vi "viewerFrontEnd.vi"(8 "error in (no error)":errorcluster, 10 "defaultPath":path=path "D:/Data/Labview/BEC Suite/Hal/Channels/Camera/XML Camera Settings/CameraSettings.xml", 11 "CameraSettingsViewer in":refnum<class "andorSettingsViewer.lvclass">) -> (0 "error out":errorcluster, 3 "CameraSettingsViewer out":refnum<class "andorSettingsViewer.lvclass">)   [LabVIEW 2011, in "Views.lvlib" / "Camera.lvlib" / "andorSettingsViewer.lvclass"]
uses:
  andorSettingsViewer.lvclass
  Tools/Filing/FileSystem/FileSystem.lvclass
  Tools/SettingsEventManager/SettingsEventsManager.lvclass
  Tools/SettingsViewer/settingsViewer.lvclass
panel:
  in  "save Current Settings":bool
  in  "Close Settings Mananger":bool
  in  "Load Current Settings":bool
  in  "Load Settings From File":path
  in  "Tab Control":T1(tab)=enum."shift_speeds"
  in  "acquisition_mode":u16(ring)=2 caption="Acquisition Mode" items=["Single Shot"=1, "Accumulative Series"=2, "Kinetic Series"=3, "Fast Kinetic Series"=4, "Run 'till Abort"=5]
  in  "readout_mode":i16(ring)=1 caption="Readout Mode" items=["Full Vertical Binning"=0, "Single Track"=3, "Multi-Track"=1, "Random Track"=2, "Full Resolusion Image"=4]
  in  "subArea_coordinate":i32(listbox) caption="ROI Coordinates of \nBottom left corner"
  in  "vertical_binning":dbl=1.0 caption="Vertical Binning \n(min 0)"
  in  "horizontal_binning":dbl=1.0 caption="Horizontal Binning \n(min 0)"
  in  "subArea_height":dbl=1024.0 caption="ROI and Single Track:\nROI Height"
  in  "subArea_width":dbl=1024.0 caption="ROI Width"
  in  "offset":dbl caption="Single Track:\nOffset"
  in  "number_tracks":i32 caption="Multi Track:\nNumber of Tracks"
  in  "track_positions":i32(listbox) caption="Track Positions"
  in  "fast_kinetic_shift_speed":dbl caption="Fast Kinetic Shift Speed [MHz]"
  in  "horizontal_shift_speed":enum16{"2.5", "1", "0.05"}(ring) caption="Horizontal Shift Speed [MHz]"
  in  "vertical_shift_speed":T2(ring)=enum."44.975" caption="Vertical Shift Speed [mus]"
  in  "fast_kinetic_image_number":dbl=1.0 caption="Number in fast Kinetic Series"
  in  "fast_kinetic_cycle_time":dbl caption="Fast Kinetic Cycle Time"
  in  "accumulative_cycle_time":dbl caption="Accumulative Cycle Time"
  in  "kinetic_cycle_time":dbl caption="Kinetic Cycle Time"
  in  "accumulation_image_number":dbl=1.0 caption="Number of Accumulations"
  in  "kinetic_image_number":dbl=1.0 caption="Number in Kinetic Series"
  in  "mode":enum16{"Automatic", "Hold Open", "Hold Closed"}(ring) caption="Shutter Mode"
  in  "open_time":dbl=20.0 caption="Shutter Open Time"
  in  "close_time":dbl=20.0 caption="Shutter Close Time"
  in  "exposure_time":dbl=0.02 caption="Exposure Time [s]"
  out "start_trigger":string caption="Trigger Channel"
  in  "trigger_mode":u16(ring) caption="Trigger Mode" items=["Internal"=0, "External"=1, "External Start"=6]
  in  "fast_trigger":bool caption="Fast Triggering"
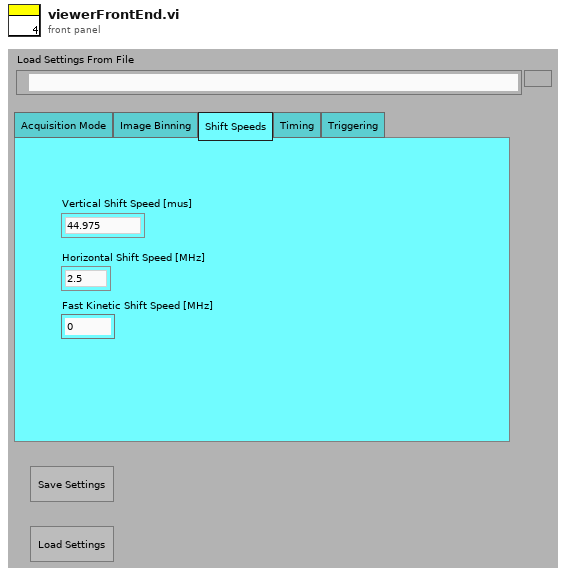
[diagram p1: front panel]
types:
  T1 = enum32{"modes", "image_binning", "shift_speeds", "timing", "triggering"}
  T2 = enum16{"0.525", "0.875", "1.575", "2.975", "5.775", "11.375", "22.575", "44.975"}
  T3 = cluster{"settingsFrontEndEvents":cluster{"loadSettingsFromPath":refnum<user-event>, "lookUpElementEvent":refnum<user-event>, "saveSettings":refnum<user-event>, "loadSettings":refnum<user-event>, "close":refnum<user-event>, "replaceElement":refnum<user-event>, "findParentNodes":refnum<user-event>, "createNode":refnum<user-event>}, "settingBackEndEvents":cluster{"defaultSettingsPathRequest":refnum<user-event>, "searchResultEvent":refnum<user-event>, "settingsSaved":refnum<user-event>, "settingsLoaded":refnum<user-event>, "foundParentNode":refnum<user-event>}}
  T4 = cluster{"loadSettingsFromPath":refnum<user-event>, "lookUpElementEvent":refnum<user-event>, "saveSettings":refnum<user-event>, "loadSettings":refnum<user-event>, "close":refnum<user-event>, "replaceElement":refnum<user-event>, "findParentNodes":refnum<user-event>, "createNode":refnum<user-event>}
  T5 = cluster{"defaultSettingsPathRequest":refnum<user-event>, "searchResultEvent":refnum<user-event>, "settingsSaved":refnum<user-event>, "settingsLoaded":refnum<user-event>, "foundParentNode":refnum<user-event>}
  T6 = enum16{"Number", "String", "NumberArray", "StringArray", "xmlNode"}
  T7 = cluster{"Label.Text":string, string, "DigDisp.Text":string}
  T8 = cluster{"Label.Text":string, string, "RingText.Text":string}
  T9 = typedef "LVPoint32TypeDef.ctl" = cluster{"Horizontal":i32, "Vertical":i32}
  T10 = typedef "LVRowAndColumnTypeDef.ctl" = cluster{"Row":i32, "Column":i32}
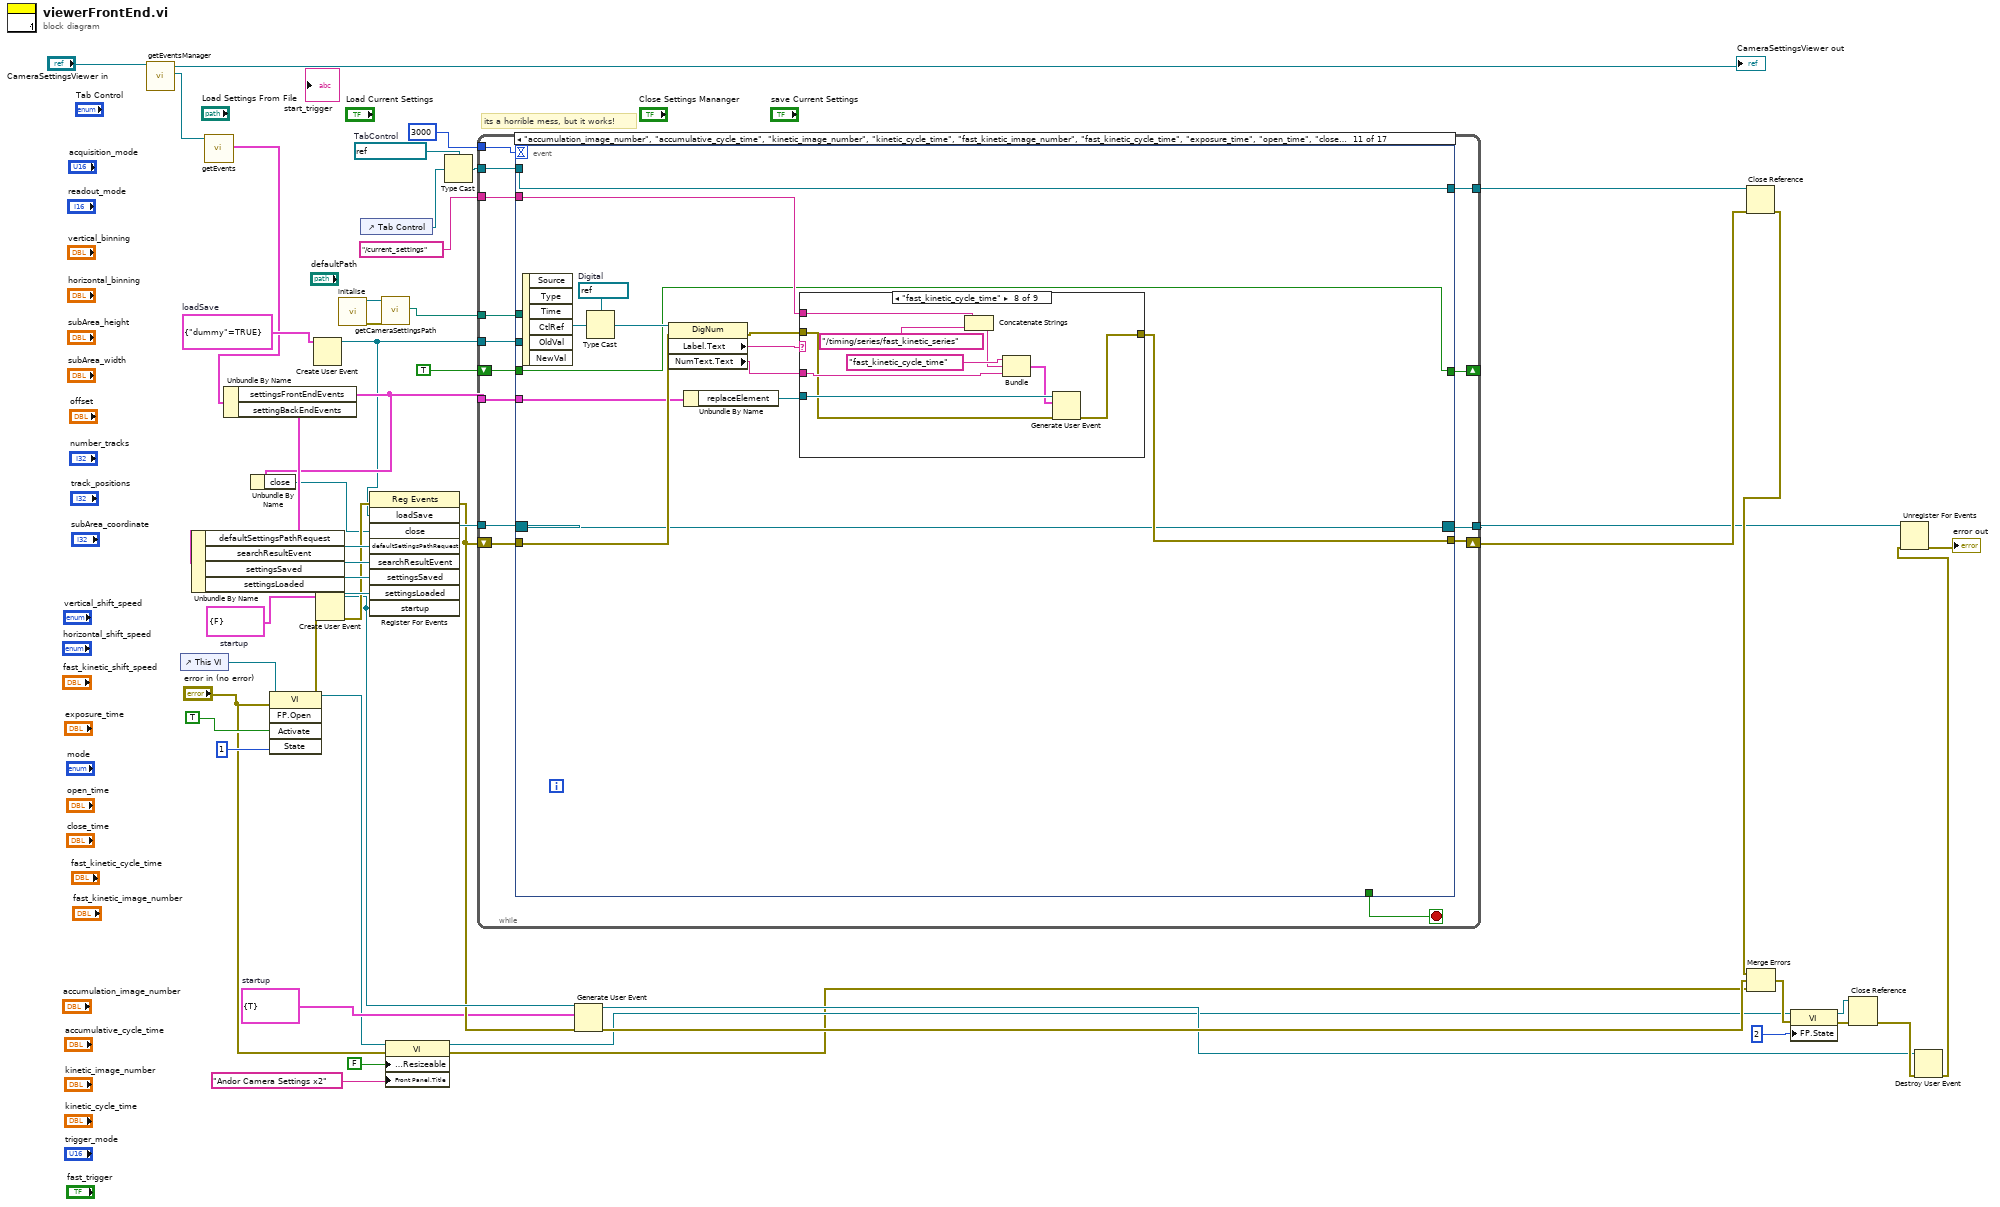
[diagram p0: block diagram]
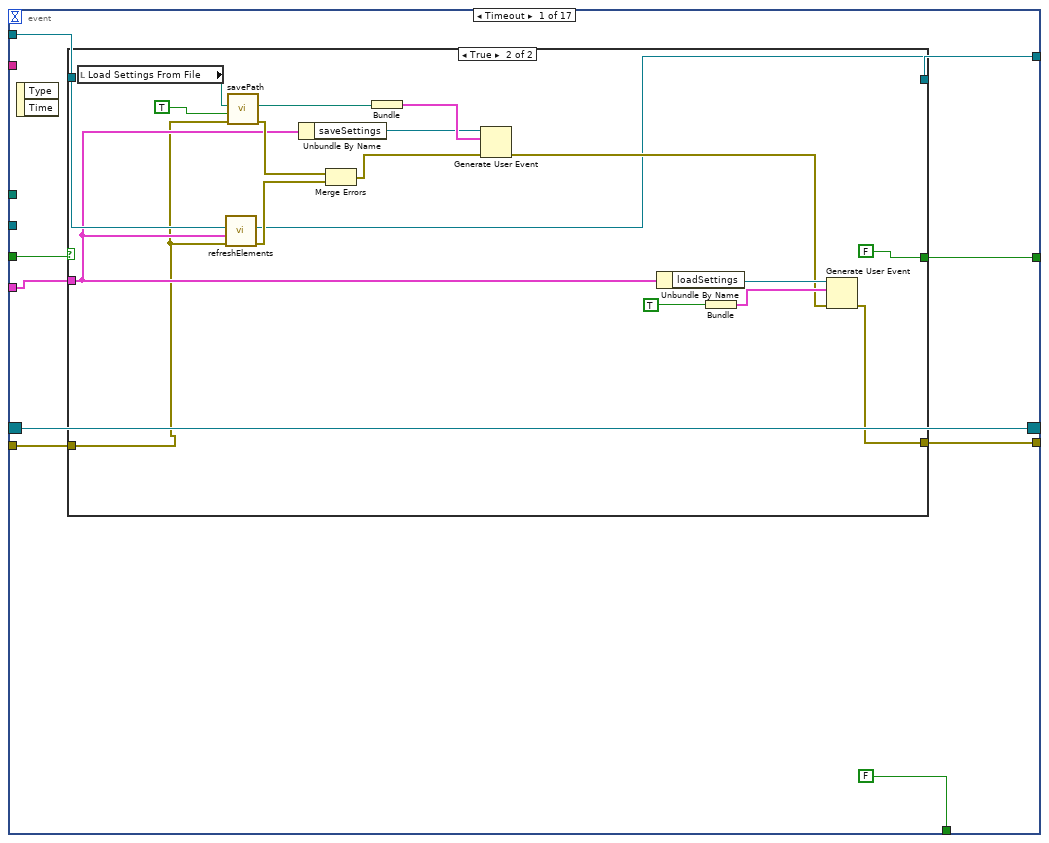
[diagram p2: hidden frame]
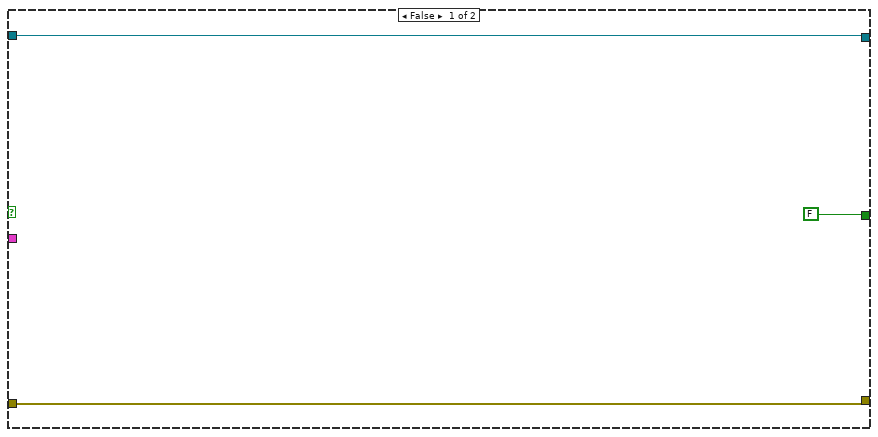
[diagram p3: hidden frame]
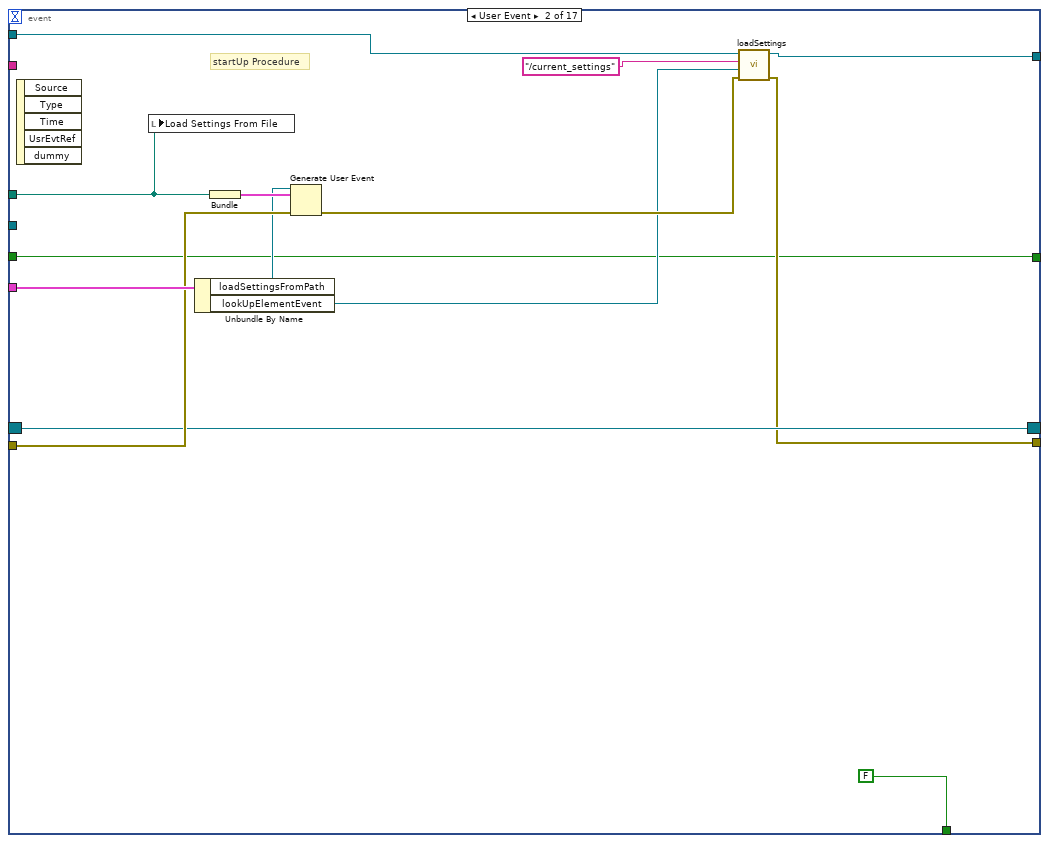
[diagram p4: hidden frame]
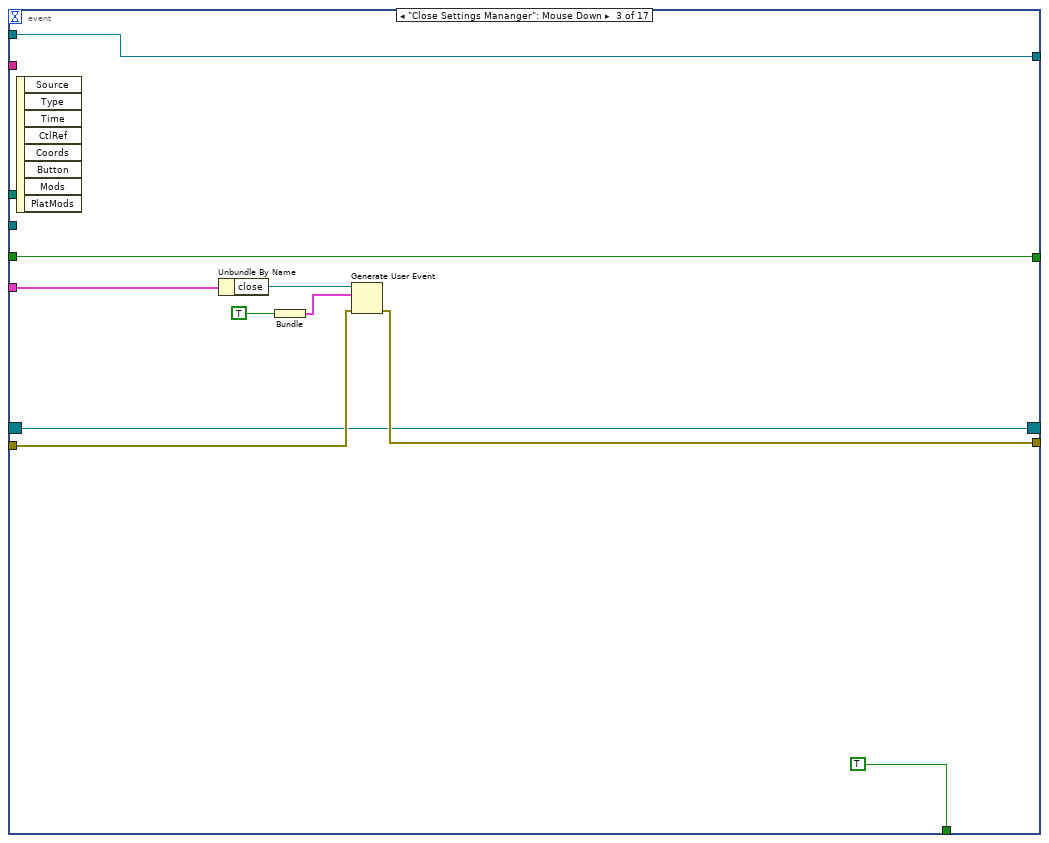
[diagram p5: hidden frame]
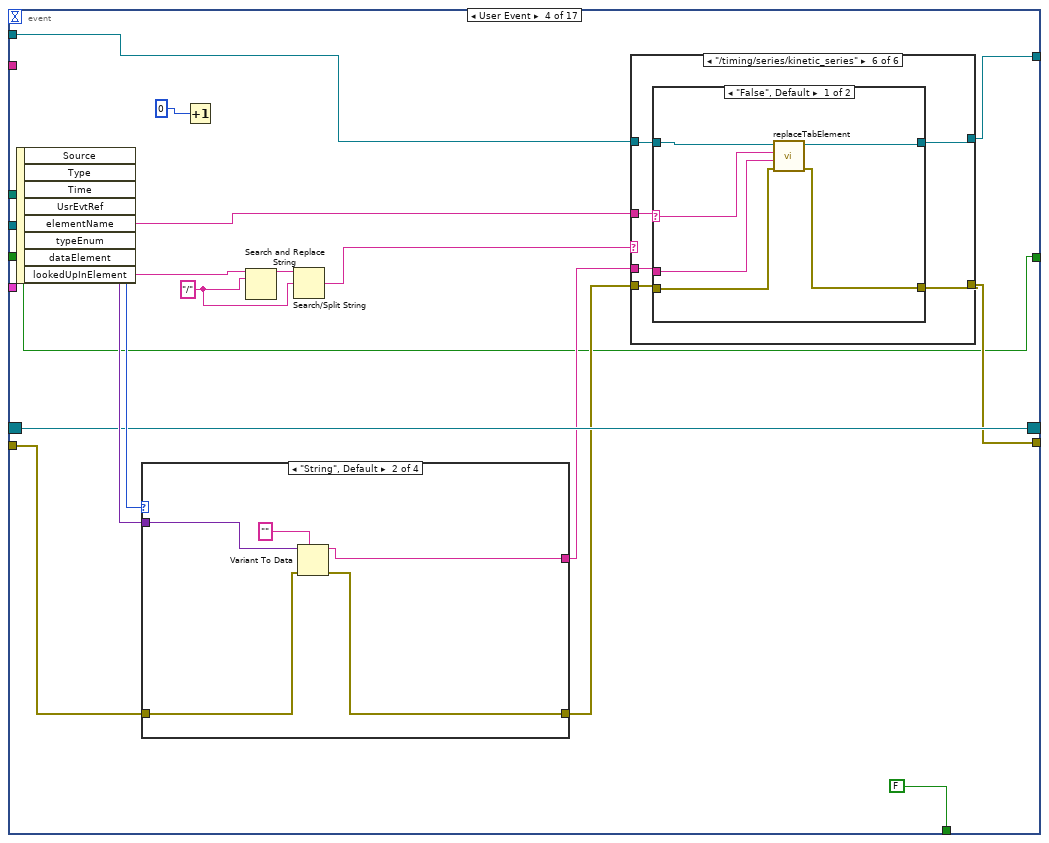
[diagram p6: hidden frame]
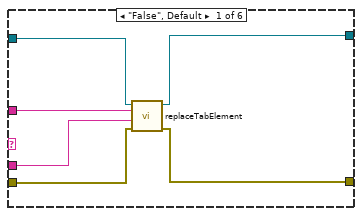
[diagram p7: hidden frame]
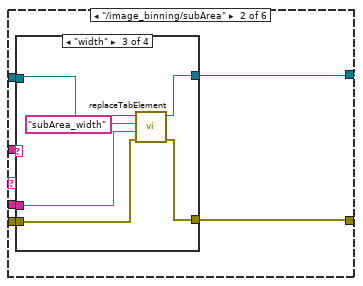
[diagram p8: hidden frame]
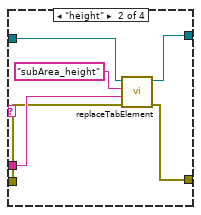
[diagram p10: hidden frame]
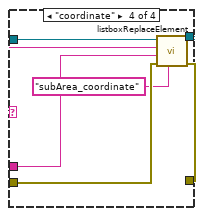
[diagram p11: hidden frame]
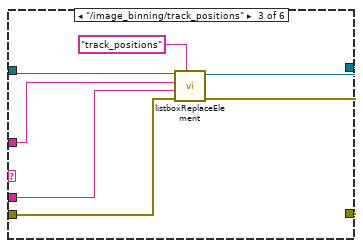
[diagram p12: hidden frame]
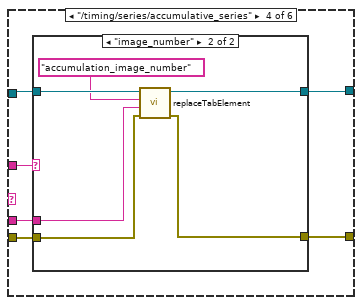
[diagram p13: hidden frame]
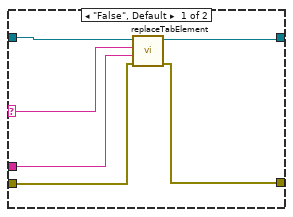
[diagram p14: hidden frame]
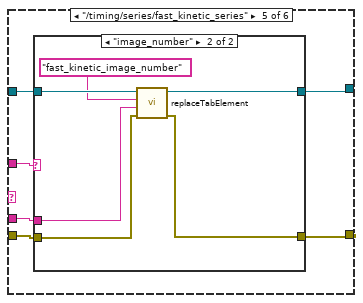
[diagram p15: hidden frame]
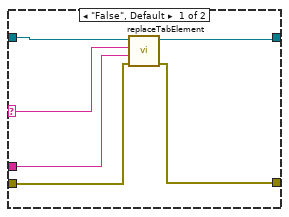
[diagram p16: hidden frame]
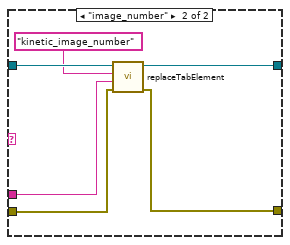
[diagram p17: hidden frame]
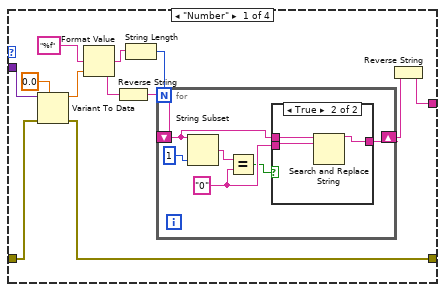
[diagram p18: hidden frame]
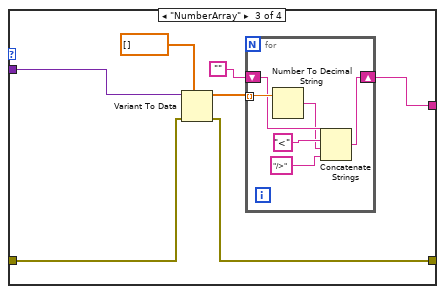
[diagram p20: hidden frame]
diagram:
  w12 = cluster{"dummy":bool} {"dummy"=TRUE}  # loadSave
  w22 = refnum<vi> refnum  # TabControl
  w32 = cluster{"dummy":bool} {"dummy"=TRUE}  # startup
  w36 = cluster{"dummy":bool} {"dummy"=FALSE}  # startup
  # "its a horrible mess, but it works!"
  n1 = call-dynamic "getEventsManager.vi"("SettingsViewer.lvclass in"="CameraSettingsViewer in") -> ("Tools.lvlib:Settings.lvlib:SettingsEventsManager.lvclass"=w8:refnum<class "SettingsEventsManager.lvclass">, "SettingsViewer.lvclass out"=→"CameraSettingsViewer out":refnum<class "andorSettingsViewer.lvclass">)  [unwired: 8 in, 1 out]
  n2 = control-ref of="This VI"() -> (w43:refnum<vi>)
  n3 = call-dynamic "getEvents.vi"("SettingsEventsManager in"=w8) -> ("settingsEvents"=w7:T3)  [unwired: 8 in, 2 out]
  n4 = Unbundle By Name(w7) -> ("settingsFrontEndEvents"=w14:T4, "settingBackEndEvents"=w51:T5)
  n5 = Unbundle By Name(w51) -> ("defaultSettingsPathRequest"=w50:refnum<user-event>, "searchResultEvent"=w49:refnum<user-event>, "settingsSaved"=w48:refnum<user-event>, "settingsLoaded"=w47:refnum<user-event>)
  n6 = Unbundle By Name(w14) -> ("close"=w13:refnum<user-event>)
  n7 = invoke class="VI" method="FP.Open"(reference=w43, error in="error in (no error)", "Activate"=TRUE, "State"=1) -> (reference out=w19:refnum<vi>, error out=w35:errorcluster)  [unwired: 1 in, 3 out]
  n8 = Create User Event(user event datatype=w12) -> (user event=w11:refnum<user-event>)  [unwired: 1 in, 1 out]
  n9 = Create User Event(user event datatype=w36, error in=w35) -> (user event=w34:refnum<user-event>, error out=w37:errorcluster)
  n10 = call "initalise.vi"() -> ("error out"=w4:errorcluster, "FileSystem out"=w5:refnum<class "FileSystem.lvclass">)  [unwired: 10 in]
  n11 = control-ref of="Tab Control"() -> (w23:refnum<vi>)
  n12 = register-events(error in=w37, w11, w13, w50, w49, w48, w47, w34) -> (reference out=w44:refnum<event-registration>, error out=w33:errorcluster)  [unwired: 1 in]
  n13 = call-dynamic "getCameraSettingsPath.vi"("error in (no error)"=w4, "FileSystem.lvclass in"=w5) -> ("CameraSettingsPath"=w6:path)  [unwired: 7 in, 2 out]
  n14 = property class="VI"(reference=w19, error in="error in (no error)", "Front Panel.Resizeable"=FALSE, "Front Panel.Title"="Andor Camera Settings x2") -> (reference out=w16:refnum<vi>, error out=w15:errorcluster)
  n15 = Type Cast(type=w22, x=w23) -> (*(type *) &x=w20:refnum<vi>)
  n16 = while {
    tunnel: w14 -> [w65]
    shift-right: [w62] -> w45
    shift-left: w33 -> [w64]
    tunnel: "/current_settings" -> [w61]
    tunnel: w6 -> [w60]
    tunnel: w44 -> [w56]
    tunnel: [w59] -> w29
    tunnel: [w58] -> w21
    tunnel: w20 -> [w57]
    tunnel: w11 -> [w55]
    tunnel: 3000 -> [w54]
    shift-right: [w52] -> _
    shift-left: TRUE -> [w53]
    stop <- w63 stop-if-true
    n17 = event shown="[10] \"accumulation_image_number\", \"accumulative_cycle_time\", \"kinetic_image_number\", \"kinetic_cycle_time\", \"fast_kinetic_image_number\", \"fast_kinetic_cycle_time\", \"exposure_time\", \"open_time\", \"close_time\": Value Change" {
      selector: w56 -> [w73 w106 w112 w133 w291 _ w328 w353 w364 w398 w434 w530 w556 w580 w610 _ w640]
      dyn-events: [w73 w106 w112 w133 w291 _ w328 w353 w364 w398 w434 w530 w556 w580 w610 _ w640] -> w59
      timeout: w54 -> [_ _ _ _ _ _ _ _ _ _ _ _ _ _ _ _ _]
      tunnel: w65 -> [w71 w109 w118 _ w289 w311 w315 w351 w365 w397 w440 w533 _ w586 w616 w631 _]
      tunnel: w64 -> [w70 w108 w114 w134 w292 w307 w318 w343 w366 w402 w443 w531 w546 w569 w613 w636 w641]
      tunnel: [FALSE FALSE TRUE FALSE FALSE _ _ FALSE _ _ _ _ _ _ _ _ TRUE] -> w63
      tunnel: [w68 w99 w113 w123 w286 w308 w329 w348 w355 w396 w435 w529 w545 w576 w611 w639 w641] -> w62
      tunnel: w61 -> [_ _ _ _ _ _ _ w338 w363 w407 w437 w539 _ w578 w623 _ _]
      tunnel: [w69 w102 w111 w124 w287 w309 w321 w344 w361 w399 w433 w528 w544 w568 w609 w632 w643] -> w58
      tunnel: w60 -> [_ w97 _ _ _ _ _ _ _ _ _ _ _ _ _ _ _]
      tunnel: w57 -> [w72 w103 w111 w122 w288 w310 w322 w344 w361 w399 w433 w528 w544 w570 w609 w637 w643]
      tunnel: w55 -> [_ _ _ _ _ _ _ _ _ _ _ _ _ _ _ _ _]
      tunnel: w53 -> [w67 w96 w110 w120 w282 w306 w314 w333 w354 w395 w432 w527 w543 w557 w608 w626 w642]
      tunnel: [w66 w96 w110 w120 w282 w306 w314 w333 w354 w395 w432 w527 w543 w557 w608 w626 w642] -> w52
      event Timeout {
        n18 = event-data() -> ()  [unwired: 1 in, 2 out]
        n19 = case shown="True" w67 {
          tunnel: w72 -> [w76 w84]
          tunnel: w71 -> [_ w83]
          tunnel: w70 -> [w77 w82]
          tunnel: [w76 w80] -> w69
          tunnel: [w77 w79] -> w68
          tunnel: [FALSE FALSE] -> w66
          frame False {
          }
          frame True {
            n20 = local read "Load Settings From File"() -> (w81:path)
            n21 = call "refreshElements.vi"("error in (no error)"=w82, "settingsFrontEndEvents"=w83, "Tab ref in"=w84) -> ("error out"=w91:errorcluster, "Tab ref out"=w80:refnum<vi>)  [unwired: 7 in]
            n22 = call "savePath.vi"("error in (no error)"=w82, "overwrite?"=TRUE, "Path  in"=w81) -> ("error out"=w92:errorcluster, "Path out"=w85:path)  [unwired: 6 in, 1 out]
            n23 = Unbundle By Name(w83) -> ("saveSettings"=w88:refnum<user-event>)
            n24 = Merge Errors(w92, w91) -> (w90:errorcluster)
            n25 = Bundle("Path out"=w85) -> (w89:cluster{"Path out":path})  [unwired: 1 in]
            n26 = Generate User Event(user event=w88, event data cluster=w89, error in=w90) -> (error out=w87:errorcluster)  [unwired: 1 out]
            n27 = Unbundle By Name(w83) -> ("loadSettings"=w95:refnum<user-event>)
            n28 = Bundle(TRUE) -> (w93:cluster{bool})  [unwired: 1 in]
            n29 = Generate User Event(user event=w95, event data cluster=w93, error in=w87) -> (error out=w79:errorcluster)  [unwired: 1 out]
          }
        }
      }
      event User Event {
        # "startUp Procedure"
        n30 = event-data() -> ()  [unwired: 1 in, 5 out]
        n31 = local write "Load Settings From File"(w97) -> ()
        n32 = Unbundle By Name(w109) -> ("loadSettingsFromPath"=w104:refnum<user-event>, "lookUpElementEvent"=w98:refnum<user-event>)
        n33 = Bundle("CameraSettingsPath"=w97) -> (w105:cluster{"CameraSettingsPath":path})  [unwired: 1 in]
        n34 = Generate User Event(user event=w104, event data cluster=w105, error in=w108) -> (error out=w100:errorcluster)  [unwired: 1 out]
        n35 = call "loadSettings.vi"("error in (no error)"=w100, "lookUpElementEvent"=w98, "whichSettings"="/current_settings", "TabCtl Refnum in"=w103) -> ("error out"=w99:errorcluster, "TabCtl Refnum out"=w102:refnum<vi>)  [unwired: 6 in]
      }
      event "Close Settings Mananger": Mouse Down {
        n36 = event-data() -> ()  [unwired: 1 in, 8 out]
        n37 = Unbundle By Name(w118) -> ("close"=w117:refnum<user-event>)
        n38 = Bundle(TRUE) -> (w115:cluster{bool})  [unwired: 1 in]
        n39 = Generate User Event(user event=w117, event data cluster=w115, error in=w114) -> (error out=w113:errorcluster)  [unwired: 1 out]
      }
      event User Event {
        w128 = "/"
        n40 = event-data() -> ("elementName"=w131:string, "typeEnum"=w136:T6, "dataElement"=w135:variant, "lookedUpInElement"=w129:string)  [unwired: 1 in, 4 out]
        n41 = case shown="\"String\", Default" w136 {
          tunnel: w135 -> [w238 w256 w262 w276]
          tunnel: w134 -> [w239 w255 w261 w275]
          tunnel: [w240 w254 w260 w270] -> w125
          tunnel: [w232 w252 w257 w271] -> w126
          frame "Number" {
            n42 = Variant To Data(error in=w239, type=0.0, Variant=w238) -> (data=w231:dbl, error out=w240:errorcluster)
            n43 = Format Value(format string="%f", value (0)=w231) -> (output string=w234:string)  [unwired: 1 in]
            n44 = Reverse String(1:w234) -> (0:w236:string)
            n45 = String Length(string=w234) -> (length=w235:i32)
            n46 = for {
              N: w235 -> [_]
              shift-right: [w242] -> w233
              shift-left: w236 -> [w245]
              w244 = "0"
              n47 = String Subset(string=w245, length (rest)=1) -> (substring=w246:string)  [unwired: 1 in]
              n48 = Equal?(x=w246, y=w244) -> (x = y?=w243:bool)
              n49 = case shown="True" w243 {
                tunnel: w245 -> [w248 w251]
                tunnel: w244 -> [_ w249]
                tunnel: [w248 w250] -> w242
                frame False {
                }
                frame True {
                  n50 = Search and Replace String(input string=w251, search string=w249) -> (result string=w250:string)  [unwired: 6 in, 3 out]
                }
              }
            }
            n51 = Reverse String(1:w233) -> (0:w232:string)
          }
          frame "String", Default {
            n52 = Variant To Data(error in=w255, type="", Variant=w256) -> (data=w252:string, error out=w254:errorcluster)
          }
          frame "NumberArray" {
            n53 = Variant To Data(error in=w261, type=dbl[] [], Variant=w262) -> (data=w259:dbl[], error out=w260:errorcluster)
            n54 = for {
              tunnel: w259 -> [w269] mode=indexing
              shift-right: [w264] -> w257
              shift-left: "" -> [w268]
              n55 = Number To Decimal String(number=w269) -> (decimal integer string=w266:string)  [unwired: 1 in]
              n56 = Concatenate Strings(w268, "<", w266, "/>") -> (w264:string)
            }
          }
          frame "StringArray" {
            n57 = Variant To Data(error in=w275, type=string[] [], Variant=w276) -> (data=w273:string[], error out=w270:errorcluster)
            n58 = for {
              shift-right: [w277] -> w271
              shift-left: "" -> [w278]
              tunnel: w273 -> [w279] mode=indexing
              n59 = Concatenate Strings(w278, "<", w279, "/>") -> (w277:string)
            }
          }
        }
        n60 = Increment(x=0) -> ()  [unwired: 1 out]
        n61 = Search and Replace String(input string=w129, search string=w128) -> (result string=w130:string)  [unwired: 6 in, 3 out]
        n62 = Search/Split String(string=w130, search string/char (-)=w128) -> (match + rest of string=w127:string)  [unwired: 1 in, 2 out]
        n63 = case shown="\"/timing/series/kinetic_series\"" w127 {
          tunnel: w131 -> [w141 w143 w174 w180 w198 w216]
          tunnel: w122 -> [w142 w144 w176 w182 w200 w218]
          tunnel: w126 -> [w140 w148 w173 w181 w199 w217]
          tunnel: w125 -> [w139 w147 w171 w177 w195 w213]
          tunnel: [w138 w146 w170 w178 w196 w214] -> w123
          tunnel: [w137 w145 w175 w179 w197 w215] -> w124
          frame "False", Default {
            n64 = call "replaceTabElement.vi"("error in (no error)"=w139, "replaceWith"=w140, "replaceElementLabeled"=w141, "Tab ref in"=w142) -> ("error out"=w138:errorcluster, "Tab ref out"=w137:refnum<vi>)  [unwired: 6 in]
          }
          frame "/image_binning/subArea" {
            n65 = case shown="\"width\"" w143 {
              selector: w143 -> [_ _ _ w164]
              tunnel: w148 -> [_ w156 w158 w165]
              tunnel: w147 -> [w149 w155 w159 w167]
              tunnel: [w149 w154 w160 w166] -> w146
              tunnel: [w150 w153 w161 w168] -> w145
              tunnel: w144 -> [w150 w152 w162 w169]
              frame "False", Default {
              }
              frame "height" {
                n66 = call "replaceTabElement.vi"("error in (no error)"=w155, "replaceWith"=w156, "replaceElementLabeled"="subArea_height", "Tab ref in"=w152) -> ("error out"=w154:errorcluster, "Tab ref out"=w153:refnum<vi>)  [unwired: 6 in]
              }
              frame "width" {
                n67 = call "replaceTabElement.vi"("error in (no error)"=w159, "replaceWith"=w158, "replaceElementLabeled"="subArea_width", "Tab ref in"=w162) -> ("error out"=w160:errorcluster, "Tab ref out"=w161:refnum<vi>)  [unwired: 6 in]
              }
              frame "coordinate" {
                n68 = call "listboxReplaceElement.vi"("inElement"="subArea_coordinate", "error in (no error)"=w167, "replaceElementWith"=w165, "elementName"=w164, "TabCtl Refnum"=w169) -> ("error out"=w166:errorcluster, "TabCtl Refnum out"=w168:refnum<vi>)  [unwired: 5 in]
              }
            }
          }
          frame "/image_binning/track_positions" {
            n69 = call "listboxReplaceElement.vi"("inElement"="track_positions", "error in (no error)"=w171, "replaceElementWith"=w173, "elementName"=w174, "TabCtl Refnum"=w176) -> ("error out"=w170:errorcluster, "TabCtl Refnum out"=w175:refnum<vi>)  [unwired: 5 in]
          }
          frame "/timing/series/accumulative_series" {
            n70 = case shown="\"image_number\"" w180 {
              selector: w180 -> [w187 _]
              tunnel: w182 -> [w188 w194]
              tunnel: w181 -> [w186 w193]
              tunnel: [w183 w191] -> w179
              tunnel: [w184 w190] -> w178
              tunnel: w177 -> [w185 w189]
              frame "False", Default {
                n71 = call "replaceTabElement.vi"("error in (no error)"=w185, "replaceWith"=w186, "replaceElementLabeled"=w187, "Tab ref in"=w188) -> ("error out"=w184:errorcluster, "Tab ref out"=w183:refnum<vi>)  [unwired: 6 in]
              }
              frame "image_number" {
                n72 = call "replaceTabElement.vi"("error in (no error)"=w189, "replaceWith"=w193, "replaceElementLabeled"="accumulation_image_number", "Tab ref in"=w194) -> ("error out"=w190:errorcluster, "Tab ref out"=w191:refnum<vi>)  [unwired: 6 in]
              }
            }
          }
          frame "/timing/series/fast_kinetic_series" {
            n73 = case shown="\"image_number\"" w198 {
              selector: w198 -> [w205 _]
              tunnel: w200 -> [w206 w212]
              tunnel: w199 -> [w204 w211]
              tunnel: [w201 w209] -> w197
              tunnel: [w202 w208] -> w196
              tunnel: w195 -> [w203 w207]
              frame "False", Default {
                n74 = call "replaceTabElement.vi"("error in (no error)"=w203, "replaceWith"=w204, "replaceElementLabeled"=w205, "Tab ref in"=w206) -> ("error out"=w202:errorcluster, "Tab ref out"=w201:refnum<vi>)  [unwired: 6 in]
              }
              frame "image_number" {
                n75 = call "replaceTabElement.vi"("error in (no error)"=w207, "replaceWith"=w211, "replaceElementLabeled"="fast_kinetic_image_number", "Tab ref in"=w212) -> ("error out"=w208:errorcluster, "Tab ref out"=w209:refnum<vi>)  [unwired: 6 in]
              }
            }
          }
          frame "/timing/series/kinetic_series" {
            n76 = case shown="\"False\", Default" w216 {
              selector: w216 -> [w223 _]
              tunnel: w218 -> [w224 w230]
              tunnel: w217 -> [w222 w229]
              tunnel: [w219 w227] -> w215
              tunnel: [w220 w226] -> w214
              tunnel: w213 -> [w221 w225]
              frame "False", Default {
                n77 = call "replaceTabElement.vi"("error in (no error)"=w221, "replaceWith"=w222, "replaceElementLabeled"=w223, "Tab ref in"=w224) -> ("error out"=w220:errorcluster, "Tab ref out"=w219:refnum<vi>)  [unwired: 6 in]
              }
              frame "image_number" {
                n78 = call "replaceTabElement.vi"("error in (no error)"=w225, "replaceWith"=w229, "replaceElementLabeled"="kinetic_image_number", "Tab ref in"=w230) -> ("error out"=w226:errorcluster, "Tab ref out"=w227:refnum<vi>)  [unwired: 6 in]
              }
            }
          }
        }
      }
      event "Load Settings From File": Value Change {
        n79 = event-data() -> ()  [unwired: 1 in, 6 out]
        n80 = local read "Load Settings From File"() -> (w283:path)
        n81 = Equal?(x=path "", y=w283) -> (x = y?=w285:bool)
        n82 = case shown="False" w285 {
          tunnel: w292 -> [w302 w305]
          tunnel: w283 -> [w301 _]
          tunnel: w289 -> [w299 _]
          tunnel: w288 -> [w298 w304]
          tunnel: [w297 w304] -> w287
          tunnel: [w294 w305] -> w286
          frame False {
            n83 = Unbundle By Name(w299) -> ("lookUpElementEvent"=w296:refnum<user-event>, "loadSettingsFromPath"=w303:refnum<user-event>)
            n84 = Bundle("Load Settings From File"=w301) -> (w300:cluster{"Load Settings From File":path})  [unwired: 1 in]
            n85 = Generate User Event(user event=w303, event data cluster=w300, error in=w302) -> (error out=w295:errorcluster)  [unwired: 1 out]
            n86 = call "loadSettings.vi"("error in (no error)"=w295, "lookUpElementEvent"=w296, "whichSettings"="/current_settings", "TabCtl Refnum in"=w298) -> ("error out"=w294:errorcluster, "TabCtl Refnum out"=w297:refnum<vi>)  [unwired: 6 in]
          }
          frame True {
          }
        }
      }
      event User Event {
        n87 = event-data() -> ()  [unwired: 1 in, 5 out]
        n88 = Unbundle By Name(w311) -> ("lookUpElementEvent"=w313:refnum<user-event>)
        n89 = call "loadSettings.vi"("error in (no error)"=w307, "lookUpElementEvent"=w313, "whichSettings"="/current_settings", "TabCtl Refnum in"=w310) -> ("error out"=w308:errorcluster, "TabCtl Refnum out"=w309:refnum<vi>)  [unwired: 6 in]
      }
      event "Load Current Settings": Mouse Down {
        n90 = event-data() -> ()  [unwired: 1 in, 8 out]
        n91 = local read "Load Settings From File"() -> (w319:path)
        n92 = call "refreshElements.vi"("error in (no error)"=w318, "settingsFrontEndEvents"=w315, "Tab ref in"=w322) -> ("error out"=w326:errorcluster, "Tab ref out"=w321:refnum<vi>)  [unwired: 7 in]
        n93 = call "savePath.vi"("error in (no error)"=w318, "overwrite?"=TRUE, "Path  in"=w319) -> ("error out"=w327:errorcluster, "Path out"=w316:path)  [unwired: 6 in, 1 out]
        n94 = Unbundle By Name(w315) -> ("saveSettings"=w323:refnum<user-event>)
        n95 = Merge Errors(w327, w326) -> (w325:errorcluster)
        n96 = local write "Load Settings From File"(w316) -> ()
        n97 = Bundle("Path out"=w316) -> (w324:cluster{"Path out":path})  [unwired: 1 in]
        n98 = Generate User Event(user event=w323, event data cluster=w324, error in=w325) -> (error out=w320:errorcluster)  [unwired: 1 out]
        n99 = Unbundle By Name(w315) -> ("loadSettings"=w332:refnum<user-event>)
        n100 = Bundle(TRUE) -> (w330:cluster{bool})  [unwired: 1 in]
        n101 = Generate User Event(user event=w332, event data cluster=w330, error in=w320) -> (error out=w329:errorcluster)  [unwired: 1 out]
      }
      event "acquisition_mode", "readout_mode", "trigger_mode": Value Change {
        w346 = refnum<vi> refnum  # Ring
        n102 = event-data() -> ("CtlRef"=w345:refnum<vi>)  [unwired: 1 in, 5 out]
        n103 = Unbundle By Name(w351) -> ("replaceElement"=w350:refnum<user-event>)
        n104 = Type Cast(type=w346, x=w345) -> (*(type *) &x=w347:refnum<vi>)
        n105 = property class="Ring"(reference=w347, error in=w343) -> (error out=w342:errorcluster, "Label.Text"=w340:string, "DigDisp.Text"=w334:string)  [unwired: 1 out]
        n106 = Equal?(x="trigger_mode", y=w340) -> (x = y?=w339:bool)
        n107 = Concatenate Strings(w338, "/triggering") -> (w336:string)
        n108 = Select(t=w336, s=w339, f=w338) -> (s? t:f=w335:string)
        n109 = Bundle("Label.Text"=w340, w335, "DigDisp.Text"=w334) -> (w349:T7)  [unwired: 1 in]
        n110 = Generate User Event(user event=w350, event data cluster=w349, error in=w342) -> (error out=w348:errorcluster)  [unwired: 1 out]
      }
      event "vertical_binning", "horizontal_binning", "subArea_height", "subArea_width", "offset": Value Change {
        w368 = refnum<vi> refnum  # Digital
        n111 = event-data() -> ("CtlRef"=w367:refnum<vi>)  [unwired: 1 in, 5 out]
        n112 = Unbundle By Name(w365) -> ("replaceElement"=w357:refnum<user-event>)
        n113 = Type Cast(type=w368, x=w367) -> (*(type *) &x=w369:refnum<vi>)
        n114 = property class="DigNum"(reference=w369, error in=w366) -> (error out=w356:errorcluster, "Label.Text"=w360:string, "NumText.Text"=w358:string)  [unwired: 1 out]
        n115 = Concatenate Strings(w363, "/image_binning") -> (w359:string)
        n116 = case shown="\"subArea_height\"" w360 {
          selector: w360 -> [w375 _ _]
          tunnel: [w376 w381 w390] -> w355
          tunnel: w359 -> [w374 w379 w389]
          tunnel: w358 -> [w373 w380 w388]
          tunnel: w357 -> [w371 w378 w387]
          tunnel: w356 -> [w370 w377 w386]
          frame "False", Default {
            n117 = Bundle(w375, w374, "NumText.Text"=w373) -> (w372:cluster{string, string, "NumText.Text":string})  [unwired: 1 in]
            n118 = Generate User Event(user event=w371, event data cluster=w372, error in=w370) -> (error out=w376:errorcluster)  [unwired: 1 out]
          }
          frame "subArea_height" {
            n119 = Concatenate Strings(w379, "/subArea") -> (w383:string)
            n120 = Bundle("height", w383, "NumText.Text"=w380) -> (w382:cluster{string, string, "NumText.Text":string})  [unwired: 1 in]
            n121 = Generate User Event(user event=w378, event data cluster=w382, error in=w377) -> (error out=w381:errorcluster)  [unwired: 1 out]
          }
          frame "subArea_width" {
            n122 = Concatenate Strings(w389, "/subArea") -> (w392:string)
            n123 = Bundle("width", w392, "NumText.Text"=w388) -> (w391:cluster{string, string, "NumText.Text":string})  [unwired: 1 in]
            n124 = Generate User Event(user event=w387, event data cluster=w391, error in=w386) -> (error out=w390:errorcluster)  [unwired: 1 out]
          }
        }
      }
      event "vertical_shift_speed", "horizontal_shift_speed", "fast_kinetic_shift_speed": Value Change {
        n125 = event-data() -> ("CtlRef"=w405:refnum<vi>)  [unwired: 1 in, 5 out]
        n126 = property class="Num"(reference=w405, error in=w402) -> (reference out=w403:refnum<vi>, error out=w401:errorcluster, "Label.Text"=w404:string)
        n127 = Concatenate Strings(w407, "/shift_speeds") -> (w400:string)
        n128 = case shown="\"False\", Default" w404 {
          selector: w404 -> [w414 w427]
          tunnel: w403 -> [w419 w431]
          tunnel: w401 -> [w416 w428]
          tunnel: w400 -> [w413 w426]
          tunnel: w397 -> [w415 w424]
          tunnel: [w408 w420] -> w396
          frame "False", Default {
            w418 = refnum<vi> refnum  # Enum
            n129 = Type Cast(type=w418, x=w419) -> (*(type *) &x=w417:refnum<vi>)
            n130 = Unbundle By Name(w415) -> ("replaceElement"=w412:refnum<user-event>)
            n131 = property class="Enum"(reference=w417, error in=w416) -> (error out=w409:errorcluster, "RingText.Text"=w410:string)  [unwired: 1 out]
            n132 = Bundle(w414, w413, "RingText.Text"=w410) -> (w411:cluster{string, string, "RingText.Text":string})  [unwired: 1 in]
            n133 = Generate User Event(user event=w412, event data cluster=w411, error in=w409) -> (error out=w408:errorcluster)  [unwired: 1 out]
          }
          frame "fast_kinetic_shift_speed" {
            w430 = refnum<vi> refnum  # Digital
            n134 = Type Cast(type=w430, x=w431) -> (*(type *) &x=w429:refnum<vi>)
            n135 = Unbundle By Name(w424) -> ("replaceElement"=w423:refnum<user-event>)
            n136 = property class="DigNum"(reference=w429, error in=w428) -> (error out=w421:errorcluster, "NumText.Text"=w425:string)  [unwired: 1 out]
            n137 = Bundle(w427, w426, "NumText.Text"=w425) -> (w422:cluster{string, string, "NumText.Text":string})  [unwired: 1 in]
            n138 = Generate User Event(user event=w423, event data cluster=w422, error in=w421) -> (error out=w420:errorcluster)  [unwired: 1 out]
          }
        }
      }
      event "accumulation_image_number", "accumulative_cycle_time", "kinetic_image_number", "kinetic_cycle_time", "fast_kinetic_image_number", "fast_kinetic_cycle_time", "exposure_time", "open_time", "close_time": Value Change {
        w445 = refnum<vi> refnum  # Digital
        n139 = event-data() -> ("CtlRef"=w442:refnum<vi>)  [unwired: 1 in, 5 out]
        n140 = Type Cast(type=w445, x=w442) -> (*(type *) &x=w444:refnum<vi>)
        n141 = property class="DigNum"(reference=w444, error in=w443) -> (error out=w441:errorcluster, "Label.Text"=w438:string, "NumText.Text"=w436:string)  [unwired: 1 out]
        n142 = Unbundle By Name(w440) -> ("replaceElement"=w439:refnum<user-event>)
        n143 = case shown="\"fast_kinetic_cycle_time\"" w438 {
          selector: w438 -> [w452 w461 w470 _ _ _ _ _ _]
          tunnel: w439 -> [w449 w458 w467 w481 w490 w499 w508 w517 w526]
          tunnel: [w446 w455 w464 w476 w485 w494 w503 w511 w520] -> w435
          tunnel: w437 -> [w454 w463 w472 w480 w489 w498 w507 w516 w525]
          tunnel: w441 -> [w447 w456 w465 w474 w483 w492 w501 w509 w519]
          tunnel: w436 -> [w450 w459 w468 w475 w484 w493 w500 w510 w518]
          frame "exposure_time", Default {
            n144 = Concatenate Strings(w454, "/timing") -> (w451:string)
            n145 = Bundle(w452, w451, "NumText.Text"=w450) -> (w448:cluster{string, string, "NumText.Text":string})  [unwired: 1 in]
            n146 = Generate User Event(user event=w449, event data cluster=w448, error in=w447) -> (error out=w446:errorcluster)  [unwired: 1 out]
          }
          frame "open_time" {
            n147 = Concatenate Strings(w463, "/timing/shutter_timing") -> (w460:string)
            n148 = Bundle(w461, w460, "NumText.Text"=w459) -> (w457:cluster{string, string, "NumText.Text":string})  [unwired: 1 in]
            n149 = Generate User Event(user event=w458, event data cluster=w457, error in=w456) -> (error out=w455:errorcluster)  [unwired: 1 out]
          }
          frame "close_time" {
            n150 = Concatenate Strings(w472, "/timing/shutter_timing") -> (w469:string)
            n151 = Bundle(w470, w469, "NumText.Text"=w468) -> (w466:cluster{string, string, "NumText.Text":string})  [unwired: 1 in]
            n152 = Generate User Event(user event=w467, event data cluster=w466, error in=w465) -> (error out=w464:errorcluster)  [unwired: 1 out]
          }
          frame "accumulation_image_number" {
            n153 = Concatenate Strings(w480, "/timing/series/accumulative_series") -> (w477:string)
            n154 = Bundle("image_number", w477, "NumText.Text"=w475) -> (w473:cluster{string, string, "NumText.Text":string})  [unwired: 1 in]
            n155 = Generate User Event(user event=w481, event data cluster=w473, error in=w474) -> (error out=w476:errorcluster)  [unwired: 1 out]
          }
          frame "accumulative_cycle_time" {
            n156 = Concatenate Strings(w489, "/timing/series/accumulative_series") -> (w486:string)
            n157 = Bundle("accumulative_cycle_time", w486, "NumText.Text"=w484) -> (w482:cluster{string, string, "NumText.Text":string})  [unwired: 1 in]
            n158 = Generate User Event(user event=w490, event data cluster=w482, error in=w483) -> (error out=w485:errorcluster)  [unwired: 1 out]
          }
          frame "kinetic_image_number" {
            n159 = Concatenate Strings(w498, "/timing/series/kinetic_series") -> (w495:string)
            n160 = Bundle("image_number", w495, "NumText.Text"=w493) -> (w491:cluster{string, string, "NumText.Text":string})  [unwired: 1 in]
            n161 = Generate User Event(user event=w499, event data cluster=w491, error in=w492) -> (error out=w494:errorcluster)  [unwired: 1 out]
          }
          frame "kinetic_cycle_time" {
            n162 = Concatenate Strings(w507, "/timing/series/kinetic_series") -> (w504:string)
            n163 = Bundle("kinetic_cycle_time", w504, "NumText.Text"=w500) -> (w502:cluster{string, string, "NumText.Text":string})  [unwired: 1 in]
            n164 = Generate User Event(user event=w508, event data cluster=w502, error in=w501) -> (error out=w503:errorcluster)  [unwired: 1 out]
          }
          frame "fast_kinetic_cycle_time" {
            n165 = Concatenate Strings(w516, "/timing/series/fast_kinetic_series") -> (w513:string)
            n166 = Bundle("fast_kinetic_cycle_time", w513, "NumText.Text"=w510) -> (w512:cluster{string, string, "NumText.Text":string})  [unwired: 1 in]
            n167 = Generate User Event(user event=w517, event data cluster=w512, error in=w509) -> (error out=w511:errorcluster)  [unwired: 1 out]
          }
          frame "fast_kinetic_image_number" {
            n168 = Concatenate Strings(w525, "/timing/series/fast_kinetic_series") -> (w522:string)
            n169 = Bundle("image_number", w522, "NumText.Text"=w518) -> (w521:cluster{string, string, "NumText.Text":string})  [unwired: 1 in]
            n170 = Generate User Event(user event=w526, event data cluster=w521, error in=w519) -> (error out=w520:errorcluster)  [unwired: 1 out]
          }
        }
      }
      event "mode": Value Change {
        w537 = refnum<vi> refnum  # Enum
        n171 = event-data() -> ("CtlRef"=w538:refnum<vi>)  [unwired: 1 in, 5 out]
        n172 = Type Cast(type=w537, x=w538) -> (*(type *) &x=w536:refnum<vi>)
        n173 = property class="Enum"(reference=w536) -> ("Label.Text"=w535:string, "RingText.Text"=w534:string)  [unwired: 1 in, 2 out]
        n174 = Unbundle By Name(w533) -> ("replaceElement"=w532:refnum<user-event>)
        n175 = Concatenate Strings(w539, "/timing/shutter_timing") -> (w541:string)
        n176 = Bundle("Label.Text"=w535, w541, "RingText.Text"=w534) -> (w540:T8)  [unwired: 1 in]
        n177 = Generate User Event(user event=w532, event data cluster=w540, error in=w531) -> (error out=w529:errorcluster)  [unwired: 1 out]
      }
      event "track_positions": Mouse Down {
        n178 = event-data() -> ("CtlRef"=w547:refnum<vi>, "Coords"=w548:T9)  [unwired: 1 in, 6 out]
        n179 = property class="MCListbox (strict)"(reference=w547, error in=w546, "CellBG"=u32 16448250) -> (reference out=w551:refnum<vi>, error out=w550:errorcluster)
        n180 = invoke class="MCListbox (strict)" method="Point To Row Column"(reference=w551, error in=w550, "Point"=w548) -> (reference out=w554:refnum<vi>, error out=w549:errorcluster, "CellPosition"=w555:T10)  [unwired: 4 in, 4 out]
        n181 = property class="MCListbox (strict)"(reference=w554, error in=w549, "ActiveCell"=w555, "CellBG"=u32 9286656) -> (error out=w545:errorcluster)  [unwired: 1 out]
      }
      event "number_tracks": Value Change {
        w565 = refnum<vi> refnum  # MulticolumnListbox
        n182 = event-data() -> ("CtlRef"=w571:refnum<vi>, "OldVal"=w559:i32, "NewVal"=w563:i32)  [unwired: 1 in, 3 out]
        n183 = call "findTabElement.vi"("error in (no error)"=w569, "replaceElementLabeled"="track_positions", "Tab ref in"=w570) -> ("error out"=w564:errorcluster, "Tab Control"=w566:refnum<vi>, "Tab ref out"=w568:refnum<vi>)  [unwired: 5 in, 1 out]
        n184 = Type Cast(type=w565, x=w566) -> (*(type *) &x=w567:refnum<vi>)
        n185 = property class="DigNum (strict)"(reference=w571, error in=w564) -> (error out=w561:errorcluster, "Value"=w584:i32, "Label.Text"=w583:string)  [unwired: 1 out]
        n186 = Less?(x=w559, y=w563) -> (x < y?=w575:bool)
        n187 = property class="MCListbox"(reference=w567, error in=w564) -> (reference out=w572:refnum<vi>, error out=w573:errorcluster, "ItemNames"=w574:string[][])
        n188 = Concatenate Strings(w578, "/image_binning") -> (w577:string)
        n189 = Number To Decimal String(number=w584) -> (decimal integer string=w582:string)  [unwired: 1 in]
        n190 = case shown="True" w575 {
          tunnel: w563 -> [w591 w602]
          tunnel: w572 -> [w595 w605]
          tunnel: w574 -> [w592 w596]
          tunnel: [w588 w606] -> _
          tunnel: [w593 w604] -> w560
          tunnel: w573 -> [w594 w603]
          tunnel: w559 -> [_ w597]
          frame False {
            w587 = 0
            n191 = Array Subset(array=w592, index (row)=w587, length (row)=w591, index (col)=w587, length (col)=2) -> (w589:string[][])
            n192 = property class="MCListbox"(reference=w595, error in=w594, "ItemNames"=w589) -> (reference out=w588:refnum<vi>, error out=w593:errorcluster)
          }
          frame True {
            n193 = Subtract(x=w602, y=w597) -> (x-y=w601:i32)
            n194 = Initialize Array("0", w601, 2) -> (w599:string[][])
            n195 = Build Array (concatenate)(w596, w599) -> (w600:string[][])
            n196 = property class="MCListbox"(reference=w605, error in=w603, "ItemNames"=w600) -> (reference out=w606:refnum<vi>, error out=w604:errorcluster)
          }
        }
        n197 = Unbundle By Name(w586) -> ("replaceElement"=w585:refnum<user-event>)
        n198 = Bundle("Label.Text"=w583, w577, w582) -> (w581:cluster{"Label.Text":string, string, string})  [unwired: 1 in]
        n199 = Merge Errors(w561, w560) -> (w562:errorcluster)
        n200 = Generate User Event(user event=w585, event data cluster=w581, error in=w562) -> (error out=w576:errorcluster)  [unwired: 1 out]
      }
      event "fast_trigger": Value Change {
        n201 = event-data() -> ("CtlRef"=w625:refnum<vi>)  [unwired: 1 in, 5 out]
        n202 = Unbundle By Name(w616) -> ("replaceElement"=w615:refnum<user-event>)
        n203 = property class="Bool (strict)"(reference=w625, error in=w613) -> (error out=w612:errorcluster, "Label.Text"=w622:string, "Value"=w619:bool)  [unwired: 1 out]
        n204 = Select(t="on", s=w619, f="off") -> (s? t:f=w617:string)
        n205 = Concatenate Strings(w623, "/triggering") -> (w621:string)
        n206 = Bundle("Label.Text"=w622, w621, w617) -> (w614:cluster{"Label.Text":string, string, string})  [unwired: 1 in]
        n207 = Generate User Event(user event=w615, event data cluster=w614, error in=w612) -> (error out=w611:errorcluster)  [unwired: 1 out]
      }
      event "save Current Settings": Mouse Down; User Event {
        n208 = event-data() -> ()  [unwired: 1 in, 3 out]
        n209 = local read "Load Settings From File"() -> (w638:path)
        n210 = call "savePath.vi"("error in (no error)"=w636, "overwrite?"=FALSE, "Path  in"=w638) -> ("error out"=w635:errorcluster, "Path out"=w628:path)  [unwired: 6 in, 1 out]
        n211 = call "refreshElements.vi"("error in (no error)"=w636, "settingsFrontEndEvents"=w631, "Tab ref in"=w637) -> ("error out"=w634:errorcluster, "Tab ref out"=w632:refnum<vi>)  [unwired: 7 in]
        n212 = local write "Load Settings From File"(w628) -> ()
        n213 = Unbundle By Name(w631) -> ("saveSettings"=w629:refnum<user-event>)
        n214 = Merge Errors(w635, w634) -> (w633:errorcluster)
        n215 = Bundle("Path out"=w628) -> (w630:cluster{"Path out":path})  [unwired: 1 in]
        n216 = Generate User Event(user event=w629, event data cluster=w630, error in=w633) -> (error out=w639:errorcluster)  [unwired: 1 out]
      }
      event User Event {
        n217 = event-data() -> ()  [unwired: 1 in, 5 out]
      }
    }
  }
  n218 = Generate User Event(user event=w34, event data cluster=w32, error in=w33) -> (user event out=w24:refnum<user-event>, error out=w27:errorcluster)
  n219 = Close Reference(reference=w21, error in (no error)=w45) -> (error out=w31:errorcluster)
  n220 = Merge Errors(w31, w27, w15) -> (w30:errorcluster)
  n221 = property class="VI"(reference=w16, error in=w30, "FP.State"=2) -> (reference out=w41:refnum<vi>, error out=w40:errorcluster)
  n222 = Close Reference(reference=w41, error in (no error)=w40) -> (error out=w26:errorcluster)
  n223 = Destroy User Event(user event=w24, error in=w26) -> (error out=w25:errorcluster)
  n224 = Unregister For Events(event registration refnum=w29, error in=w25) -> (error out=→"error out":errorcluster)
